vi "MeasurementServer_Start.vi"(8 "error in (no error)":errorcluster, 9 "Server Address":string="localhost:50051", 10 "Server Certificate File (.crt)":path, 11 "Server Key File (.key)":path) -> (0 "error out":errorcluster, 1 "Cluster":T2, 2 "Event Registration Ref":refnum<event-registration>, 5 "Server Information":T2)   [LabVIEW 2019, in "labview-grpc-measurement-server.lvlib"]
uses:
  labview-grpc-measurement-server.lvlib
  MeasurementServer_InvokeEventData.ctl
  MeasurementServer_gRPCid.ctl
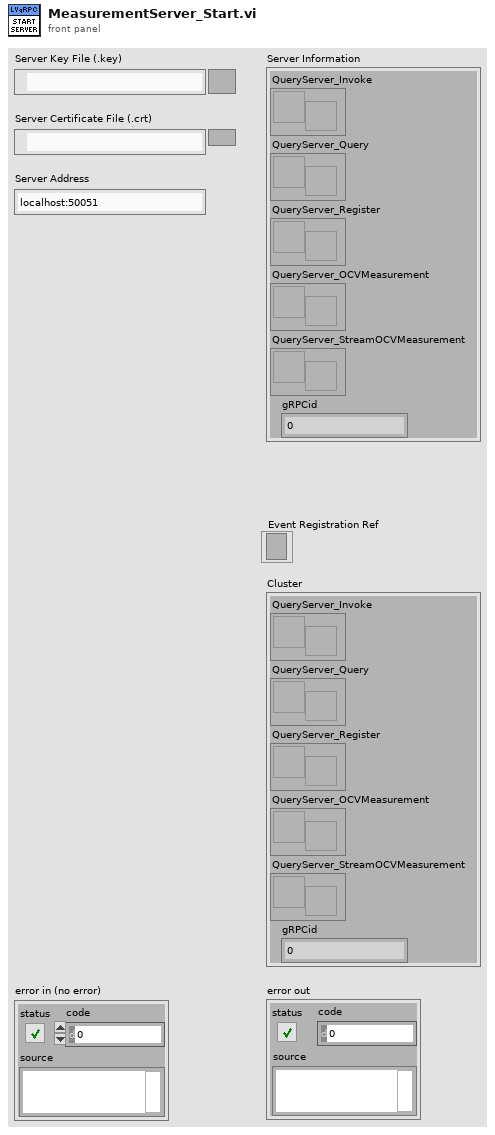
[diagram p1: front panel]
types:
  T1 = typedef "labview-grpc-measurement-server.lvlib/MeasurementServer_gRPCid.ctl" = u64
  T2 = cluster{"QueryServer_Invoke":refnum<user-event>, "QueryServer_Query":refnum<user-event>, "QueryServer_Register":refnum<user-event>, "QueryServer_OCVMeasurement":refnum<user-event>, "QueryServer_StreamOCVMeasurement":refnum<user-event>, "gRPCid":T1}
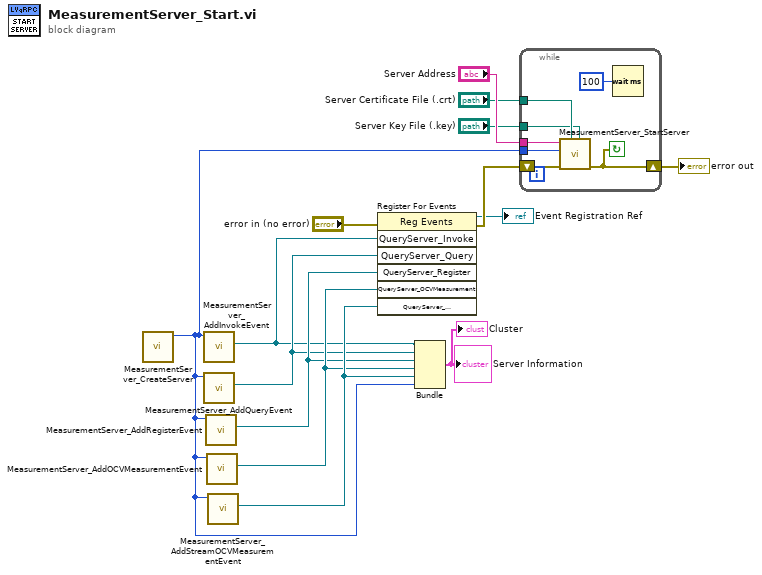
[diagram p0: block diagram]
diagram:
  n1 = call "MeasurementServer_CreateServer.vi"() -> ("gRPCid"=w14:T1)  [unwired: 11 in]
  n2 = call "MeasurementServer_AddInvokeEvent.vi"("gRPCid in"=w14) -> ("QueryServer_Invoke"=w2:refnum<user-event>)  [unwired: 9 in, 1 out]
  n3 = call "MeasurementServer_AddQueryEvent.vi"("gRPCid in"=w14) -> ("QueryServer_Query"=w3:refnum<user-event>)  [unwired: 9 in, 1 out]
  n4 = call "MeasurementServer_AddRegisterEvent.vi"("gRPCid in"=w14) -> ("QueryServer_Register"=w4:refnum<user-event>)  [unwired: 9 in, 1 out]
  n5 = call "MeasurementServer_AddOCVMeasurementEvent.vi"("gRPCid in"=w14) -> ("QueryServer_OCVMeasurement"=w5:refnum<user-event>)  [unwired: 9 in, 1 out]
  n6 = call "MeasurementServer_AddStreamOCVMeasurementEvent.vi"("gRPCid in"=w14) -> ("QueryServer_StreamOCVMeasurement"=w6:refnum<user-event>)  [unwired: 9 in, 1 out]
  n7 = register-events(error in="error in (no error)", w2, w3, w4, w5, w6) -> (reference out=→"Event Registration Ref":refnum<event-registration>, error out=w9:errorcluster)  [unwired: 1 in]
  n8 = Bundle("QueryServer_Invoke"=w2, "QueryServer_Query"=w3, "QueryServer_Register"=w4, "QueryServer_OCVMeasurement"=w5, "QueryServer_StreamOCVMeasurement"=w6, "gRPCid"=w14) -> (→"Server Information" →"Cluster":T2)  [unwired: 1 in]
  n9 = while {
    tunnel: w14 -> [w21]
    tunnel: "Server Address" -> [w20]
    tunnel: "Server Certificate File (.crt)" -> [w19]
    tunnel: "Server Key File (.key)" -> [w18]
    shift-right: [w16] -> w10
    shift-left: w9 -> [w17]
    stop <- w16 continue-if-true
    n10 = call "MeasurementServer_StartServer.vi"("Server Key File (.key)"=w18, "Server Certificate File (.crt)"=w19, "error in (no error)"=w17, "gRPCid"=w21, "Server Address"=w20) -> ("error out"=w16:errorcluster)  [unwired: 6 in]
    n11 = Wait (ms)(milliseconds to wait=u32 100) -> ()  [unwired: 1 out]
  }
  "error out" <- w10
